vi "Place New Mouse.vi"(8 "error in (no error)":errorcluster, 9 "Board Game in":refnum<class "Board Game.lvclass">, 10 "Packed refs":T1, 11 "Mouse in":refnum<class "Mouse.lvclass">) -> (0 "error out":errorcluster, 3 "Mouse out":refnum<class "Mouse.lvclass">)   [LabVIEW 2021, in "Mouse.lvclass"]
uses:
  Mouse.lvclass
  C:/Users/poche/Programs/LabVIEW/imposible snake/GameEl_class/GameEl.lvclass
  GameEl_class/private/Enum Direction.ctl
  Board Game_class/Board Game.lvclass
  Application/Packed Refs.ctl
  LVApp/Modules/Sound Manager/Typedefs/Sound Effects.ctl
  Mouse.lvclass/Mouse.ctl
  GameEl_class/GameEl.lvclass/GameEl.ctl
  <vilib>/numeric/Random Number (Range) DBL.vi
  GameEl_class/GameEl.lvclass
  Application/Application.lvclass
panel:
  out "Mouse direction":T2
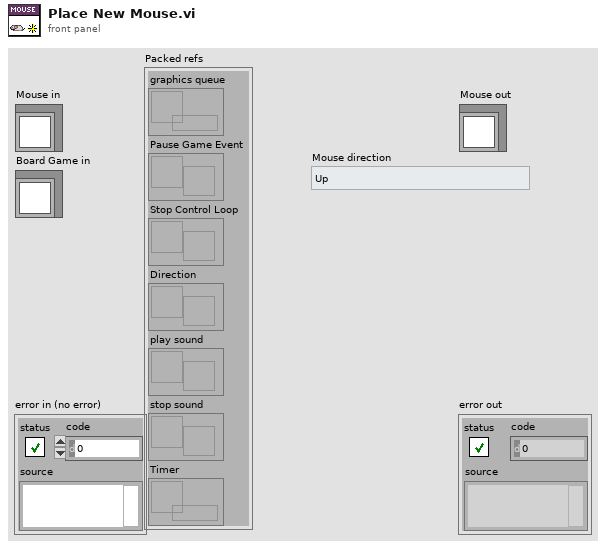
[diagram p1: front panel]
types:
  T1 = typedef "Application.lvclass/Packed Refs.ctl" = cluster{"graphics queue":refnum<queue>, "Pause Game Event":refnum<user-event>, "Stop Control Loop":refnum<user-event>, "Direction":refnum<notifier>, "play sound":refnum<user-event>, "stop sound":refnum<user-event>, "Timer":refnum<data-value>}
  T2 = typedef "GameEl.lvclass/Enum Direction.ctl" = enum16{"Up", "Down", "Forward", "Backward"}
  T3 = typedef "Sound Effects.ctl" = enum16{"Bomb In", "Bomb Out", "Bomb Touched", "Game Over", "Victory", "Eat", "10 Fruits", "Eat2", "Eat3", "Eat4", "MaxShield", "Shield", "10p", "Grape In", "Grape Out", "20p", "30p", "40p", "50p", "60p", "70p", "80p", "90p", "100p", "All shields cracked", "Mouse In", "Mouse Out", "Mouse Eaten", "Grape Eaten", "States Recover", "Broken Shield", "Bonus", "Happy Time", "explode", "Game over musica", "Back Music", "Shield Catch", "Evil lough", "Cricket In", "Cricket eaten", "Lets Go", "Jump1", "Jump2", "Jump3", "Unstoppable", "Troll Music", "winner"}
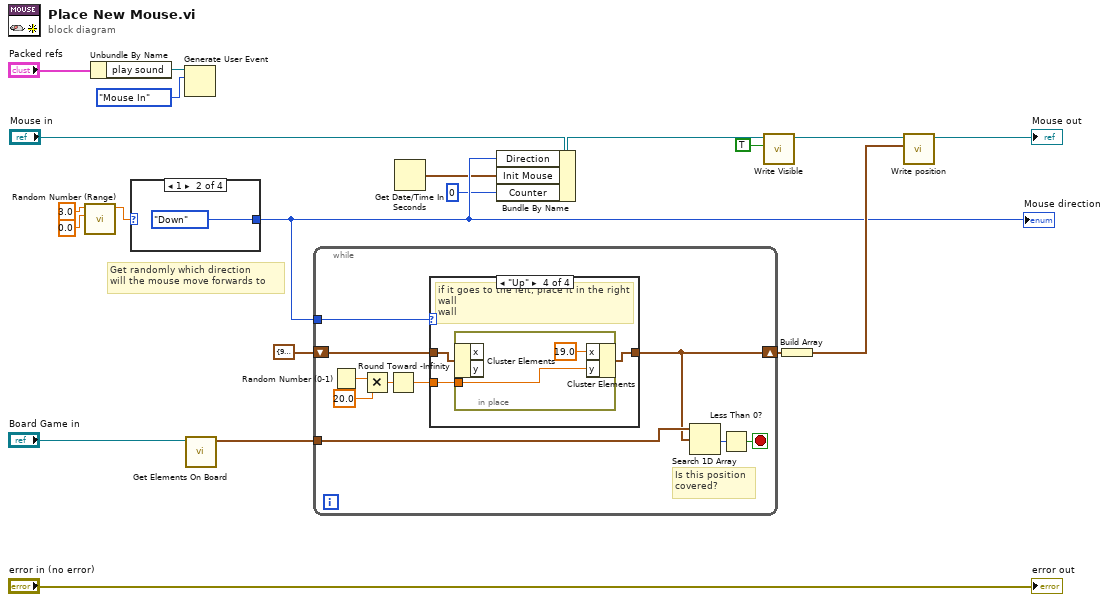
[diagram p0: block diagram]
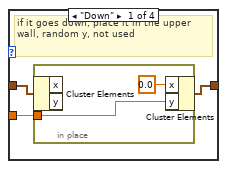
[diagram p2: hidden frame]
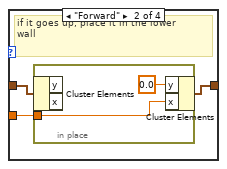
[diagram p3: hidden frame]
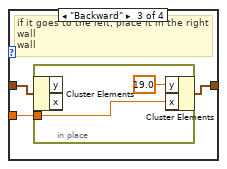
[diagram p4: hidden frame]
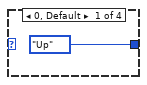
[diagram p5: hidden frame]
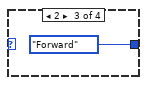
[diagram p6: hidden frame]
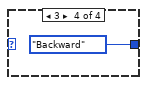
[diagram p7: hidden frame]
diagram:
  # "Get randomly which direction \nwill the mouse move forwards to"
  n1 = call-poly <vilib>:"Random Number (Range).vi"("lower bound (0)"=0.0 ("Low"), "upper bound (100)"=3.0 ("High")) -> ("number"=w17:dbl)  [unwired: 9 in]
  n2 = Unbundle By Name("Packed refs") -> ("play sound"=w2:refnum<user-event>)
  n3 = case shown="1" w17 {
    tunnel: [Enum_Direction."Up" ("Direction") Enum_Direction."Down" ("Direction") Enum_Direction."Forward" ("Direction") Enum_Direction."Backward" ("Direction")] -> w11
    frame 0, Default {
    }
    frame 1 {
    }
    frame 2 {
    }
    frame 3 {
    }
  }
  "Mouse direction" <- w11
  n4 = Generate User Event(user event=w2, event data cluster=Sound_Effects."Mouse In" ("event data")) -> ()  [unwired: 2 in, 2 out]
  n5 = call "Get Elements On Board.vi"("Board Game in"="Board Game in") -> ("position"=w5:cluster{"x":dbl, "y":dbl}[])  [unwired: 9 in, 1 out]
  n6 = while {
    tunnel: w11 -> [w33]
    shift-right: [w27] -> w10
    shift-left: cluster{"x":dbl, "y":dbl} {"x"=9.0, "y"=20.0} ("position") -> [w34]
    tunnel: w5 -> [w28]
    stop <- w25 stop-if-true
    # "Is this position \ncovered?"
    n7 = Random Number (0-1)() -> (number: 0 to 1=w32:dbl)
    n8 = Multiply(x=w32, y=20.0) -> (x*y=w31:dbl)
    n9 = Round Toward -Infinity(1:w31) -> (0:w29:dbl)
    n10 = case shown="\"Up\"" w33 {
      tunnel: w34 -> [w37 w42 w47 w52]
      tunnel: [w36 w41 w46 w51] -> w27
      tunnel: w29 -> [w35 w40 w45 w50]
      frame "Down" {
        # "if it goes down, place it in the upper \nwall, random y, not used"
        n11 = in-place {
          in-place-border: w35 -> [w38]
          n12 = in-place-cluster #1(w37) -> ()  [unwired: 2 out]
          n13 = in-place-cluster #1("x"=0.0 ("X"), "y"=w38) -> (w36:cluster{"x":dbl, "y":dbl})
        }
      }
      frame "Forward" {
        # "if it goes up, place it in the lower \nwall"
        n14 = in-place {
          in-place-border: w40 -> [w43]
          n15 = in-place-cluster #2(w42) -> ()  [unwired: 2 out]
          n16 = in-place-cluster #2("y"=0.0 ("X"), "x"=w43) -> (w41:cluster{"x":dbl, "y":dbl})
        }
      }
      frame "Backward" {
        # "if it goes to the left, place it in the right wall \nwall"
        n17 = in-place {
          in-place-border: w45 -> [w48]
          n18 = in-place-cluster #3(w47) -> ()  [unwired: 2 out]
          n19 = in-place-cluster #3("y"=19.0 ("X"), "x"=w48) -> (w46:cluster{"x":dbl, "y":dbl})
        }
      }
      frame "Up" {
        # "if it goes to the left, place it in the right wall \nwall"
        n20 = in-place {
          in-place-border: w50 -> [w53]
          n21 = in-place-cluster #4(w52) -> ()  [unwired: 2 out]
          n22 = in-place-cluster #4("x"=19.0 ("X"), "y"=w53) -> (w51:cluster{"x":dbl, "y":dbl})
        }
      }
    }
    n23 = Search 1D Array(1D array=w28, element=w27) -> (index of element=w26:i32)  [unwired: 1 in]
    n24 = Less Than 0?(x=w26) -> (x < 0?=w25:bool)
  }
  n25 = Get Date/Time In Seconds() -> (seconds since 1Jan1904=w4:timestamp)
  n26 = Bundle By Name(cluster="Mouse in", "Direction"=w11, "Init Mouse"=w4, "Counter"=u32 0) -> (w16:refnum<class "Mouse.lvclass">)
  n27 = call "Write Visible.vi"("Visible"=TRUE, "GameEl in"=w16) -> ("GameEl out"=w15:refnum<class "Mouse.lvclass">)  [unwired: 8 in, 1 out]
  n28 = Build Array(w10) -> (w12:cluster{"x":dbl, "y":dbl}[])
  n29 = call "Write position.vi"("position"=w12, "GameEl in"=w15) -> ("GameEl out"=→"Mouse out":refnum<class "Mouse.lvclass">)  [unwired: 8 in, 1 out]
  "error out" <- "error in (no error)"
